vi "Radio Buttons.vi"() -> ()   [LabVIEW 2023]
doc: "Demonstrates how to use the radio buttons control with the Value Change event."
panel:
  in  "String":string="Radio Buttons \"%s\" selected."
  in  "Stop":bool
  out "Message":string="Radio Buttons \"Option 1\" selected."
  in  "Radio Buttons":enum32{"Option 1", "Option 2", "Option 3"}(radio)
  # "Overview: Demonstrates the use of the Radio Buttons control.\nInstructions:\n1. Run the VI.\n2. Select the different options in the Radio Buttons control and observe the Message display.\n3. Click Stop to stop the VI."
  # "To add new selections to the Radio Buttons control, copy an existing selection and place it within the Radio Buttons control. Right-click the new selection and choose Visible Items > Label to change the label of the new selection, then choose the same option to hide the label again. The Boolean Text is shown on the selections because it is selectable text, whereas the label is not."
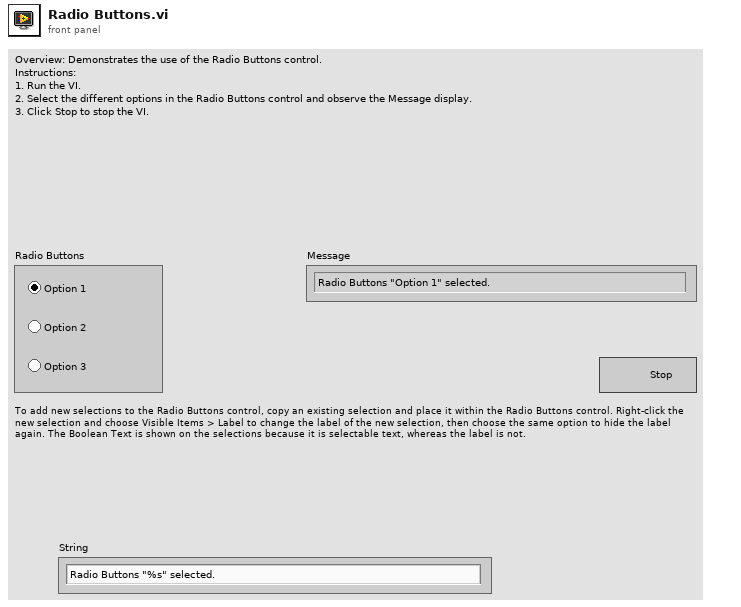
[diagram p1: front panel]
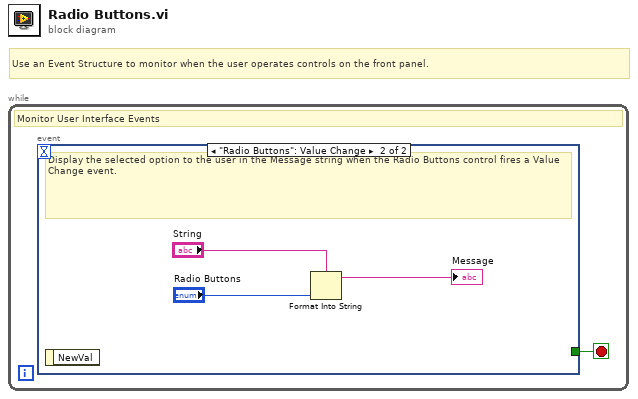
[diagram p0: block diagram]
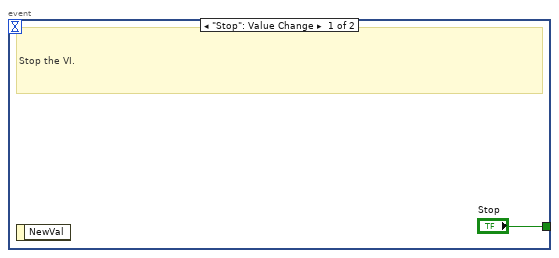
[diagram p2: hidden frame]
diagram:
  # "Use an Event Structure to monitor when the user operates controls on the front panel."
  n1 = while {
    stop <- w1 stop-if-true
    # "Monitor User Interface Events"
    n2 = event shown="[1] \"Radio Buttons\": Value Change" {
      selector: _ -> [_ _]
      dyn-events: _ -> [_ _]
      timeout: _ -> [_ _]
      tunnel: ["Stop" _] -> w1
      event "Stop": Value Change {
        # "Stop the VI."
        n3 = event-data() -> ()  [unwired: 1 in, 1 out]
      }
      event "Radio Buttons": Value Change {
        # "Display the selected option to the user in the Message string when the Radio Buttons control fires a Value Change event."
        n4 = event-data() -> ()  [unwired: 1 in, 1 out]
        n5 = Format Into String(format string="String", "Radio Buttons") -> (resulting string=→"Message":string)  [unwired: 2 in, 1 out]
      }
    }
  }
